vi "CRYLimited dB.vi"(10 "Dynamic(dB)":dbl=-40.0, 11 "Power spectrum":ext[](array[numeric]) format="%.2p") -> (3 "Limited spectrum":ext[](array[numeric]) format="%#_6p")   [LabVIEW 2013]
panel:
  out "Waveform Graph":ext[](graph)
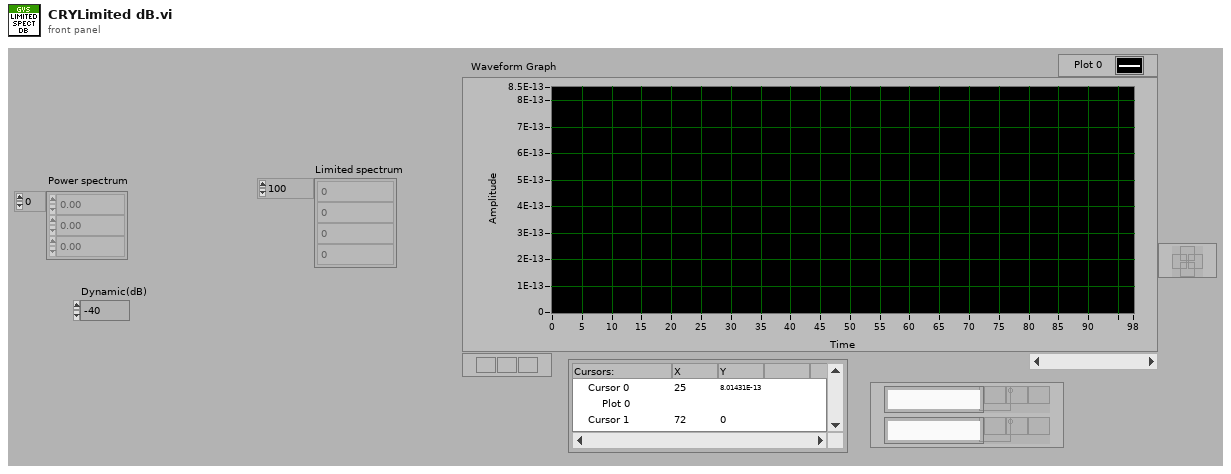
[diagram p1: front panel]
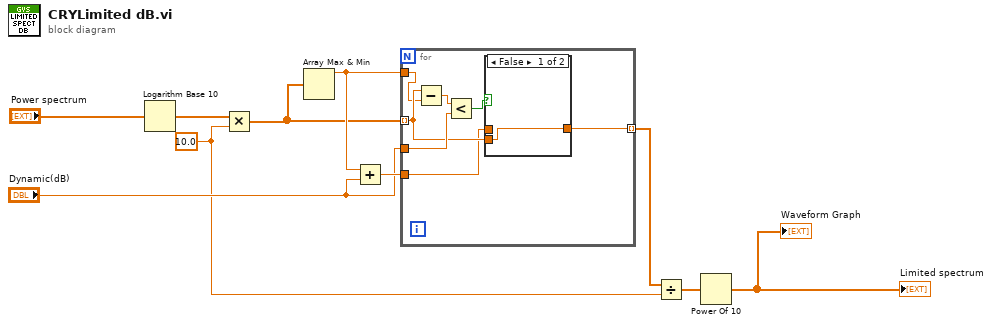
[diagram p0: block diagram]
diagram:
  w4 = 10.0 ("y")
  n1 = Logarithm Base 10(1:"Power spectrum") -> (0:w9:ext[])
  n2 = Multiply(x=w9, y=w4) -> (x*y=w3:ext[])
  n3 = Array Max & Min(array=w3) -> (max value=w8:ext)  [unwired: 3 out]
  n4 = Add(x=w8, y="Dynamic(dB)") -> (x+y=w7:ext)
  n5 = for {
    tunnel: w8 -> [w12]
    tunnel: w3 -> [w13] mode=indexing
    tunnel: "Dynamic(dB)" -> [w14]
    tunnel: [w15] -> w2 mode=indexing
    tunnel: w7 -> [w11]
    n6 = Subtract(x=w13, y=w12) -> (x-y=w17:ext)
    n7 = Less?(x=w17, y=w14) -> (x < y?=w16:bool)
    n8 = case shown="False" w16 {
      tunnel: [w18 w19] -> w15
      tunnel: w11 -> [_ w19]
      tunnel: w13 -> [w18 _]
      frame False {
      }
      frame True {
      }
    }
  }
  n9 = Divide(x=w2, y=w4) -> (x/y=w10:ext[])
  n10 = Power Of 10(x=w10) -> (10^x=→"Limited spectrum" →"Waveform Graph":ext[])
